vi "Three Ball.vi"() -> ()   [LabVIEW 2013]
uses:
  Team Code/Robot Global Data.vi
panel:
  out "Angle":dbl
  out "Distance (in)":dbl
  in  "Min. Power":dbl=0.1 format="%#_13g"
  in  "Roller / Drive Ratio":dbl=1.0
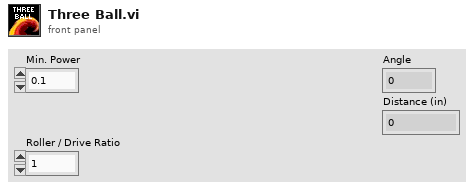
[diagram p1: front panel]
types:
  T1 = cluster{"FIRE!!!":bool, "Loader":bool, "Lock":bool, "Load":bool, "Pass":bool, "Grab":bool, "PANIC":bool, "Don't Cock":bool, "Roller Speed":dbl}
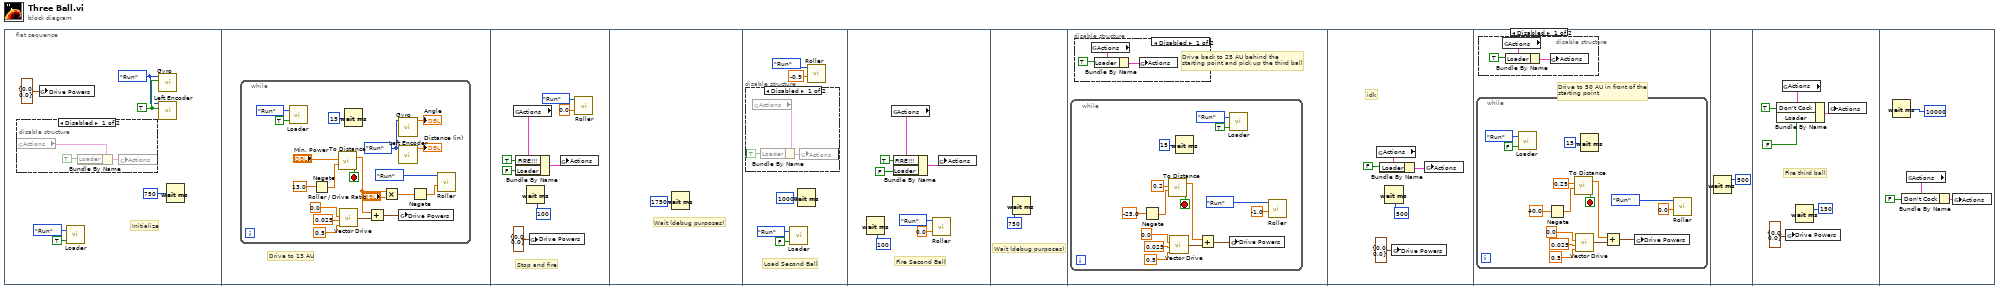
[diagram p0: block diagram]
diagram:
  n1 = flat-sequence {
    frame #0 {
      w5 = enum16{"Start", "Run", "End"}."Run" ("Enum")
      w6 = TRUE ("Reset")
      # "Initialize"
      n2 = disable-structure shown="Disabled" {
        frame Disabled {
          n3 = global read "Robot Global Data.vi" "Actions"() -> (w8:T1)
          n4 = Bundle By Name(cluster=w8, "Loader"=TRUE ("Primary Action")) -> (w9:T1)
          n5 = global write "Robot Global Data.vi" "Actions"(w9) -> ()
        }
        frame Enabled {
        }
      }
      n6 = global write "Robot Global Data.vi" "Drive Powers"(cluster{"Right":dbl, "Left":dbl} {"Right"=0.0, "Left"=0.0} ("Drive Powers")) -> ()
      n7 = call "Loader.vi"("Down (Forward)"=TRUE, "Enum"=enum16{"Start", "Run", "End"}."Run") -> ()  [unwired: 1 out]
      n8 = call "Gyro.vi"("Reset"=w6, "Enum"=w5) -> ()  [unwired: 9 in, 1 out]
      n9 = call "Left Encoder.vi"("Reset"=w6, "Enum"=w5) -> ()  [unwired: 8 in, 2 out]
      n10 = Wait (ms)(milliseconds to wait=u32 750) -> ()  [unwired: 1 out]
    }
    frame #1 {
      # "Drive to 13 AU"
      n11 = while {
        stop <- w28 stop-if-true
        w21 = enum16{"Start", "Run", "End"}."Run" ("Enum")
        n12 = call "Loader.vi"("Down (Forward)"=TRUE, "Enum"=enum16{"Start", "Run", "End"}."Run") -> ()  [unwired: 1 out]
        n13 = Negate(x=13.0) -> (-x=w19:dbl)
        n14 = call "To Distance.vi"("Destination Dist (in)"=w19, "Min. Power"="Min. Power") -> ("Reached Distance"=w28:bool, "Base Speed"=w17:dbl)  [unwired: 2 in]
        n15 = call "Vector Drive.vi"("Tolerance"=0.5, "Min. Power"=0.025, "Angle"=0.0) -> ("Motor Powers"=w24:cluster{"RMotor":dbl, "LMotor":dbl})  [unwired: 1 in]
        n16 = Wait (ms)(milliseconds to wait=u32 15) -> ()  [unwired: 1 out]
        n17 = Add(x=w17, y=w24) -> (x+y=w23:cluster{"RMotor":dbl, "LMotor":dbl})
        n18 = Multiply(x=w17, y="Roller / Drive Ratio") -> (x*y=w14:dbl)
        n19 = call "Gyro.vi"("Enum"=w21) -> ("Angle"=→"Angle":dbl)  [unwired: 10 in]
        n20 = call "Left Encoder.vi"("Enum"=w21) -> ("Distance (in)"=→"Distance (in)":dbl)  [unwired: 9 in, 1 out]
        n21 = global write "Robot Global Data.vi" "Drive Powers"(w23) -> ()
        n22 = Negate(x=w14) -> (-x=w13:dbl)
        n23 = call "Roller.vi"("Power"=w13, "Enum"=enum16{"Start", "Run", "End"}."Run") -> ()  [unwired: 2 in]
      }
    }
    frame #2 {
      # "Stop and fire"
      n24 = global read "Robot Global Data.vi" "Actions"() -> (w36:T1)
      n25 = Bundle By Name(cluster=w36, "FIRE!!!"=TRUE ("Primary Action"), "Loader"=FALSE) -> (w37:T1)
      n26 = Wait (ms)(milliseconds to wait=u32 100) -> ()  [unwired: 1 out]
      n27 = global write "Robot Global Data.vi" "Drive Powers"(cluster{"Right":dbl, "Left":dbl} {"Right"=0.0, "Left"=0.0} ("Drive Powers")) -> ()
      n28 = global write "Robot Global Data.vi" "Actions"(w37) -> ()
      n29 = call "Roller.vi"("Power"=0.0, "Enum"=enum16{"Start", "Run", "End"}."Run") -> ()  [unwired: 2 in]
    }
    frame #3 {
      # "Wait (debug purposes)"
      n30 = Wait (ms)(milliseconds to wait=u32 1750) -> ()  [unwired: 1 out]
    }
    frame #4 {
      # "Load Second Ball"
      n31 = disable-structure shown="Disabled" {
        frame Disabled {
          n32 = global read "Robot Global Data.vi" "Actions"() -> (w45:T1)
          n33 = Bundle By Name(cluster=w45, "Loader"=TRUE) -> (w46:T1)
          n34 = global write "Robot Global Data.vi" "Actions"(w46) -> ()
        }
        frame Enabled {
        }
      }
      n35 = call "Loader.vi"("Down (Forward)"=FALSE, "Enum"=enum16{"Start", "Run", "End"}."Run") -> ()  [unwired: 1 out]
      n36 = Wait (ms)(milliseconds to wait=u32 1000) -> ()  [unwired: 1 out]
      n37 = call "Roller.vi"("Power"=-0.9, "Enum"=enum16{"Start", "Run", "End"}."Run") -> ()  [unwired: 2 in]
    }
    frame #5 {
      # "Fire Second Ball"
      n38 = Wait (ms)(milliseconds to wait=u32 100) -> ()  [unwired: 1 out]
      n39 = global read "Robot Global Data.vi" "Actions"() -> (w52:T1)
      n40 = Bundle By Name(cluster=w52, "FIRE!!!"=TRUE ("Primary Action"), "Loader"=FALSE ("Primary Action")) -> (w51:T1)
      n41 = call "Roller.vi"("Power"=0.0, "Enum"=enum16{"Start", "Run", "End"}."Run") -> ()  [unwired: 2 in]
      n42 = global write "Robot Global Data.vi" "Actions"(w51) -> ()
    }
    frame #6 {
      # "Wait (debug purposes)"
      n43 = Wait (ms)(milliseconds to wait=u32 750) -> ()  [unwired: 1 out]
    }
    frame #7 {
      # "Drive back to 25 AU behind the\nstarting point and pick up the third ball"
      n44 = while {
        stop <- w72 stop-if-true
        n45 = Negate(x=-25.0) -> (-x=w66:dbl)
        n46 = call "To Distance.vi"("Destination Dist (in)"=w66, "Min. Power"=0.2) -> ("Reached Distance"=w72:bool, "Base Speed"=w64:dbl)  [unwired: 2 in]
        n47 = call "Vector Drive.vi"("Tolerance"=0.5, "Min. Power"=0.025, "Angle"=0.0) -> ("Motor Powers"=w68:cluster{"RMotor":dbl, "LMotor":dbl})  [unwired: 1 in]
        n48 = Wait (ms)(milliseconds to wait=u32 15) -> ()  [unwired: 1 out]
        n49 = Add(x=w64, y=w68) -> (x+y=w67:cluster{"RMotor":dbl, "LMotor":dbl})
        n50 = call "Loader.vi"("Down (Forward)"=TRUE, "Enum"=enum16{"Start", "Run", "End"}."Run") -> ()  [unwired: 1 out]
        n51 = global write "Robot Global Data.vi" "Drive Powers"(w67) -> ()
        n52 = call "Roller.vi"("Power"=-1.0, "Enum"=enum16{"Start", "Run", "End"}."Run") -> ()  [unwired: 2 in]
      }
      n53 = disable-structure shown="Disabled" {
        frame Disabled {
          n54 = global read "Robot Global Data.vi" "Actions"() -> (w56:T1)
          n55 = Bundle By Name(cluster=w56, "Loader"=TRUE) -> (w55:T1)
          n56 = global write "Robot Global Data.vi" "Actions"(w55) -> ()
        }
        frame Enabled {
        }
      }
    }
    frame #8 {
      # "idk"
      n57 = global read "Robot Global Data.vi" "Actions"() -> (w76:T1)
      n58 = Bundle By Name(cluster=w76, "Loader"=FALSE) -> (w77:T1)
      n59 = Wait (ms)(milliseconds to wait=u32 500) -> ()  [unwired: 1 out]
      n60 = global write "Robot Global Data.vi" "Drive Powers"(cluster{"Right":dbl, "Left":dbl} {"Right"=0.0, "Left"=0.0} ("Drive Powers")) -> ()
      n61 = global write "Robot Global Data.vi" "Actions"(w77) -> ()
    }
    frame #9 {
      # "Drive to 50 AU in front of the\nstarting point"
      n62 = while {
        stop <- w95 stop-if-true
        n63 = call "Loader.vi"("Down (Forward)"=FALSE, "Enum"=enum16{"Start", "Run", "End"}."Run") -> ()  [unwired: 1 out]
        n64 = Negate(x=40.0) -> (-x=w89:dbl)
        n65 = call "To Distance.vi"("Destination Dist (in)"=w89, "Min. Power"=0.25) -> ("Reached Distance"=w95:bool, "Base Speed"=w87:dbl)  [unwired: 2 in]
        n66 = call "Vector Drive.vi"("Tolerance"=0.5, "Min. Power"=0.025, "Angle"=0.0) -> ("Motor Powers"=w91:cluster{"RMotor":dbl, "LMotor":dbl})  [unwired: 1 in]
        n67 = Wait (ms)(milliseconds to wait=u32 15) -> ()  [unwired: 1 out]
        n68 = Add(x=w87, y=w91) -> (x+y=w90:cluster{"RMotor":dbl, "LMotor":dbl})
        n69 = global write "Robot Global Data.vi" "Drive Powers"(w90) -> ()
        n70 = call "Roller.vi"("Power"=0.0, "Enum"=enum16{"Start", "Run", "End"}."Run") -> ()  [unwired: 2 in]
      }
      n71 = disable-structure shown="Disabled" {
        frame Disabled {
          n72 = global read "Robot Global Data.vi" "Actions"() -> (w79:T1)
          n73 = Bundle By Name(cluster=w79, "Loader"=TRUE) -> (w80:T1)
          n74 = global write "Robot Global Data.vi" "Actions"(w80) -> ()
        }
        frame Enabled {
        }
      }
    }
    frame #10 {
      n75 = Wait (ms)(milliseconds to wait=u32 500) -> ()  [unwired: 1 out]
    }
    frame #11 {
      # "Fire third ball"
      n76 = global read "Robot Global Data.vi" "Actions"() -> (w102:T1)
      n77 = Bundle By Name(cluster=w102, "Don't Cock"=TRUE ("Primary Action"), "Loader"=FALSE) -> (w101:T1)
      n78 = global write "Robot Global Data.vi" "Drive Powers"(cluster{"Right":dbl, "Left":dbl} {"Right"=0.0, "Left"=0.0} ("Drive Powers")) -> ()
      n79 = Wait (ms)(milliseconds to wait=u32 150) -> ()  [unwired: 1 out]
      n80 = global write "Robot Global Data.vi" "Actions"(w101) -> ()
    }
    frame #12 {
      n81 = Wait (ms)(milliseconds to wait=u32 10000) -> ()  [unwired: 1 out]
      n82 = global read "Robot Global Data.vi" "Actions"() -> (w103:T1)
      n83 = Bundle By Name(cluster=w103, "Don't Cock"=FALSE ("Primary Action")) -> (w104:T1)
      n84 = global write "Robot Global Data.vi" "Actions"(w104) -> ()
    }
  }
